vi "Generate STM Error.vi"(5 "<append> (\"\")":string, 7 "<err> (\"\")":string, 8 "error in":errorcluster, 10 "status (T)":bool=TRUE, 11 "code":i32) -> (0 "error out":errorcluster)   [LabVIEW 2010, in "NI STM.lvlib"]
uses:
  NI STM.lvlib
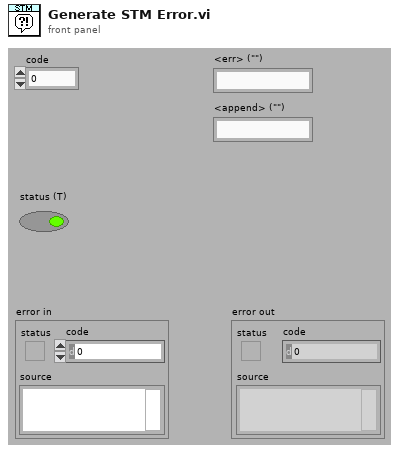
[diagram p1: front panel]
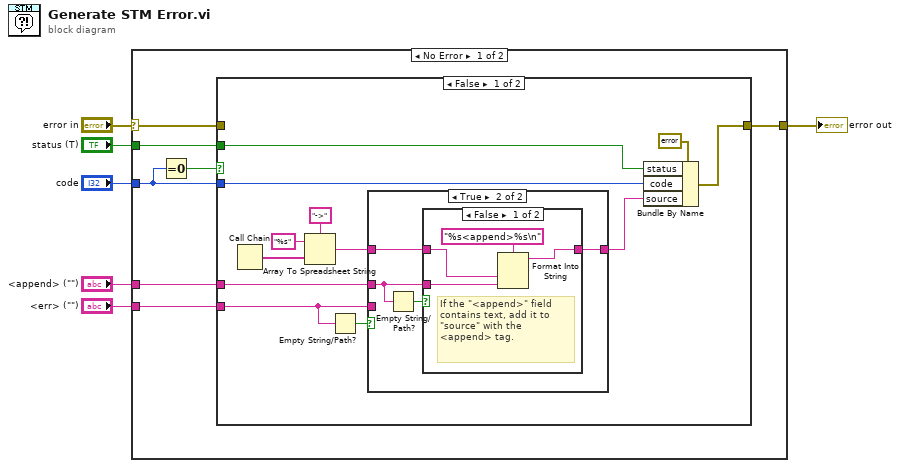
[diagram p0: block diagram]
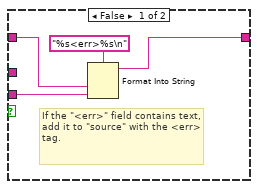
[diagram p2: hidden frame]
diagram:
  n1 = case shown="No Error" "error in" {
    selector: "error in" -> [w12 w40]
    tunnel: [w13 w40] -> w2
    tunnel: "code" -> [w11 _]
    tunnel: "<err> (\"\")" -> [w10 _]
    tunnel: "<append> (\"\")" -> [w9 _]
    tunnel: "status (T)" -> [w7 _]
    frame No Error {
      n2 = Equal To 0?(x=w11) -> (x = 0?=w8:bool)
      n3 = case shown="False" w8 {
        tunnel: w12 -> [_ w39]
        tunnel: [w25 w39] -> w13
        tunnel: w11 -> [w24 _]
        tunnel: w10 -> [w22 _]
        tunnel: w9 -> [w21 _]
        tunnel: w7 -> [w18 _]
        frame False {
          n4 = Call Chain() -> (call chain=w14:string[])
          n5 = Array To Spreadsheet String(delimiter (Tab)="->", array=w14, 3:"%s" ("format string")) -> (spreadsheet string=w15:string)
          n6 = Empty String/Path?(string/path=w22) -> (empty?=w23:bool)
          n7 = case shown="True" w23 {
            tunnel: w15 -> [w26 w31]
            tunnel: w22 -> [w27 _]
            tunnel: w21 -> [_ w32]
            tunnel: [w28 w30] -> w20
            frame False {
              # "If the \"<err>\" field contains text, add it to \"source\" with the <err> tag."
              n8 = Format Into String(format string="%s<err>%s\n", w26, w27) -> (resulting string=w28:string)  [unwired: 2 in, 1 out]
            }
            frame True {
              n9 = Empty String/Path?(string/path=w32) -> (empty?=w33:bool)
              n10 = case shown="False" w33 {
                tunnel: w32 -> [w36 _]
                tunnel: w31 -> [w37 w38]
                tunnel: [w34 w38] -> w30
                frame False {
                  # "If the \"<append>\" field contains text, add it to \"source\" with the <append> tag."
                  n11 = Format Into String(format string="%s<append>%s\n", w37, w36) -> (resulting string=w34:string)  [unwired: 2 in, 1 out]
                }
                frame True {
                }
              }
            }
          }
          n12 = Bundle By Name(cluster=errorcluster {"status"=FALSE, "code"=0, "source"=""} ("error IO"), "status"=w18, "code"=w24, "source"=w20) -> (w25:errorcluster)
        }
        frame True {
          # "Do nothing if the new code is zero."
        }
      }
    }
    frame Error {
      # "Do nothing if there is already an error on the wire."
    }
  }
  "error out" <- w2
